vi "plot_quiver.vi"(6 "Quiver Data Prealloc":dbl[][](array[numeric]), 9 "Quiver Grid":dbl[][](array[numeric]), 10 "Sensor Readings":dbl[][](array[numeric]), 11 "XYZ Gain":dbl[](array[numeric])) -> (1 "y vector":dbl[](array[numeric]), 2 "x vector":dbl[](array[numeric]), 3 "plots out":refnum<class "Base Datatype.lvclass">[](array[class]), 4 "z vector":dbl[](array[numeric]))   [LabVIEW 2016]
uses:
  <vilib>/Native 3D Graph/classes/Base Datatype.lvclass
  <vilib>/Native 3D Graph/xcontrol/3DPC_SurfacePlot.xctl
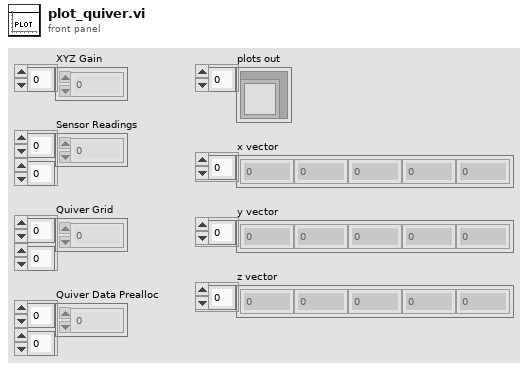
[diagram p1: front panel]
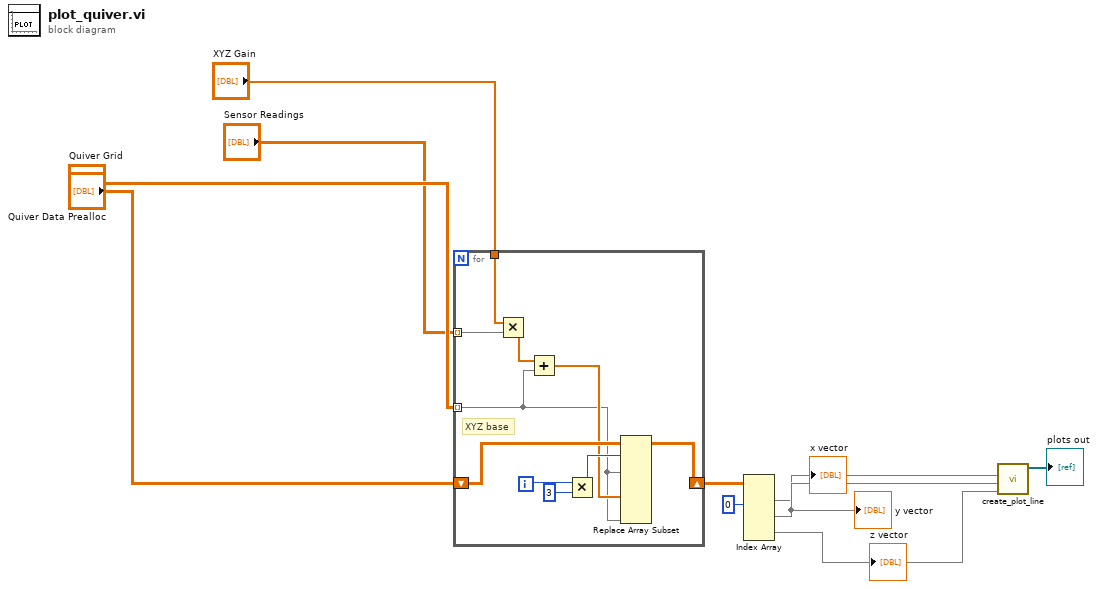
[diagram p0: block diagram]
diagram:
  n1 = for {
    tunnel: "Sensor Readings" -> [w19] mode=indexing
    tunnel: "Quiver Grid" -> [w11] mode=indexing
    tunnel: "XYZ Gain" -> [w20]
    shift-right: [w13] -> w6
    shift-left: "Quiver Data Prealloc" -> [w15]
    i -> [w17]
    # "XYZ base"
    n2 = Multiply(x=w20, y=w19) -> (x*y=w18:dbl[])
    n3 = Add(x=w18, y=w11) -> (x+y=w12:dbl[])
    n4 = Multiply(x=w17, y=3) -> (x*y=w14:i32)
    n5 = Replace Array Subset(array=w15, new element #1=w11, index (row) #1=w14, new element #2=w12, new element #3=w11) -> (w13:dbl[][])  [unwired: 5 in]
  }
  n6 = Index Array(array=w6, index (col) #1=0 ("disabled index (col)")) -> (element #1=w8:dbl[], element #2=w9:dbl[], element #3=w10:dbl[])  [unwired: 5 in]
  "x vector" <- w8
  "y vector" <- w9
  "z vector" <- w10
  n7 = call <vilib>:"create_plot_line.vi"("z vector"=w10, "y vector"=w9, "x vector"=w8) -> ("plots out"=→"plots out":refnum<class "Base Datatype.lvclass">[])  [unwired: 2 in, 6 out]
